vi "Write2LogFileAndMarkdownImage.vi"(1 "Add to log file":string, 2 "Log file before":string, 3 "Checkbox":bool, 4 "imagefilename":string) -> (0 "Log file after":string)   [LabVIEW 2019]
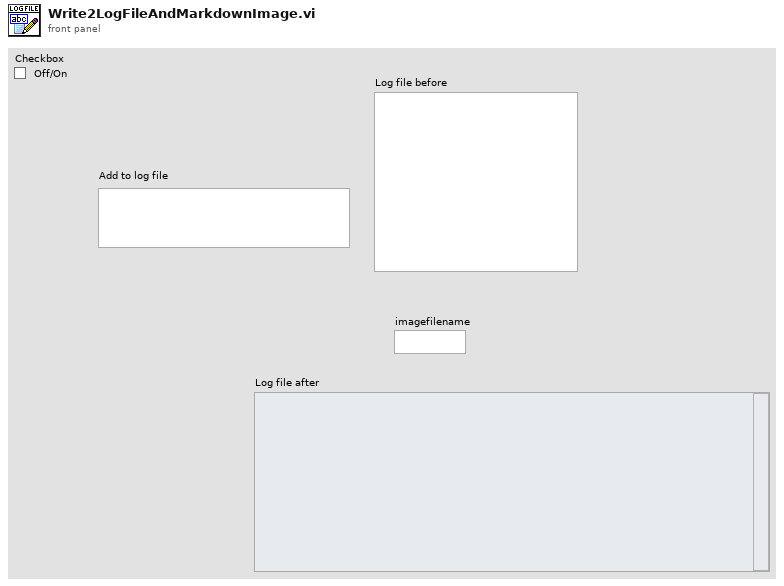
[diagram p1: front panel]
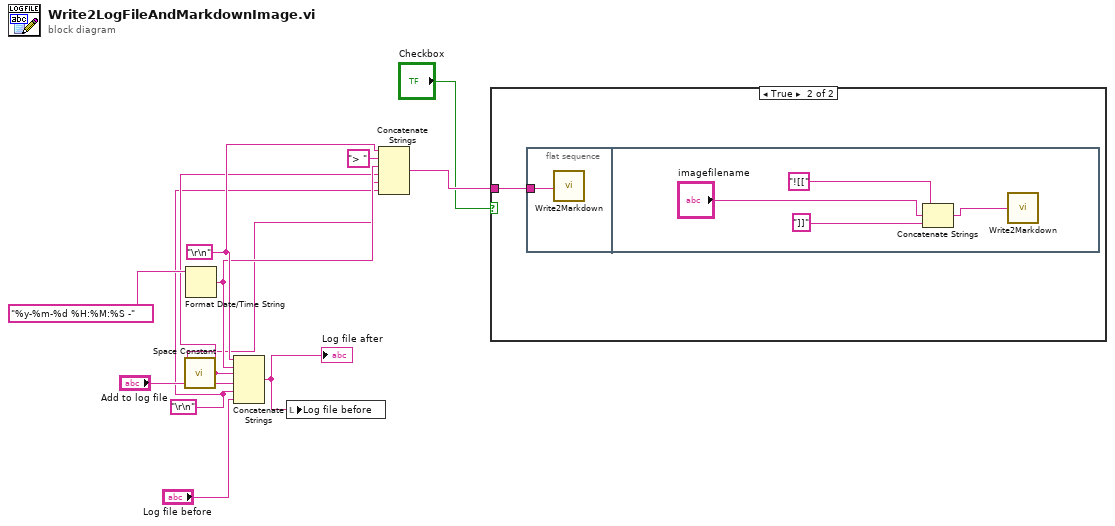
[diagram p0: block diagram]
diagram:
  w8 = "\r\n"
  w4 = "\r\n"
  n1 = call <vilib>:"Space Constant.vi"() -> ("String"=w6:string)
  n2 = Format Date/Time String(time format string (%c)="%y-%m-%d %H:%M:%S -") -> (date/time string=w7:string)  [unwired: 2 in]
  n3 = Concatenate Strings(w8, w7, w6, "Add to log file", w4, "Log file before") -> (w10:string)
  "Log file after" <- w10
  n4 = local write "Log file before"(w10) -> ()
  n5 = Concatenate Strings(w8, "> " ("string"), w7, w6, "Add to log file", w4) -> (w3:string)
  n6 = case shown="True" "Checkbox" {
    tunnel: w3 -> [_ w12]
    frame False {
    }
    frame True {
      n7 = flat-sequence {
        tunnel: w12 -> [w13]
        frame #0 {
          n8 = call "Write2Markdown.vi"("String"=w13) -> ()
        }
        frame #1 {
          n9 = Concatenate Strings("![[", "imagefilename", "]]") -> (w14:string)
          n10 = call "Write2Markdown.vi"("String"=w14) -> ()
        }
      }
    }
  }
